vi "Set In Range Trigger.vi"(7 "Trigger Direction":T2, 8 "error in (no error)":errorcluster, 10 "In Range Trigger":T1, 11 "Item Ref in":T3 format="%.0x") -> (0 "error out":errorcluster, 3 "Item Ref out":T3 format="%.0x")   [LabVIEW 2015, in "Waveform Data Logger Shared.lvlib"]
uses:
  Waveform Data Logger Shared.lvlib
  <vilib>/NI Veristand/Custom Device API/Custom Device Item Ref.ctl
  Types/Trigger Direction.ctl
  Types/In Range Trigger.ctl
  Globals/Property Strings.vi
  <vilib>/NI Veristand/Custom Device API/Set Item Property (Double).vi
  <vilib>/NI Veristand/Custom Device API/Set Item Property (Boolean).vi
  <vilib>/NI VeriStand/Custom Device API/Custom Device API.lvlib
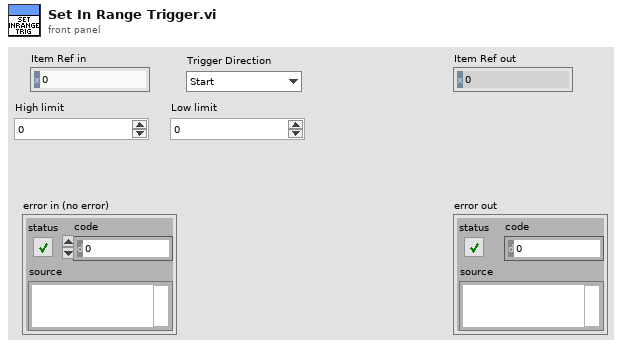
[diagram p1: front panel]
types:
  T1 = typedef "Waveform Data Logger Shared.lvlib/In Range Trigger.ctl" = cluster{"High limit":dbl, "Low limit":dbl, "Invert?":bool}
  T2 = typedef "Waveform Data Logger Shared.lvlib/Trigger Direction.ctl" = enum16{"Start", "Stop"}
  T3 = typedef "Custom Device API.lvlib/Custom Device Item Ref.ctl" = u64
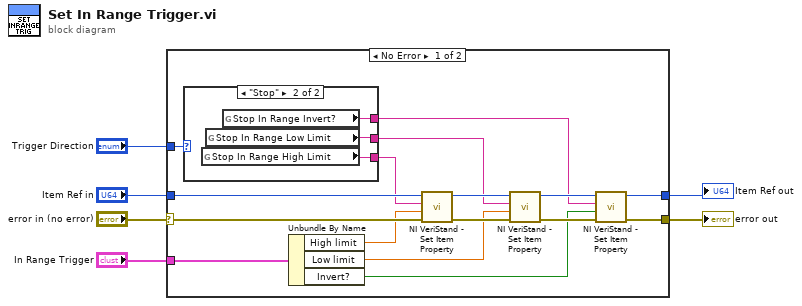
[diagram p0: block diagram]
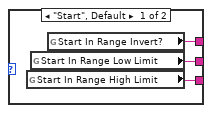
[diagram p2: hidden frame]
diagram:
  n1 = case shown="No Error" "error in (no error)" {
    selector: "error in (no error)" -> [w18 w29]
    tunnel: [w10 w30] -> w6
    tunnel: [w9 w29] -> w5
    tunnel: "Item Ref in" -> [w20 w30]
    tunnel: "In Range Trigger" -> [w19 _]
    tunnel: "Trigger Direction" -> [w17 _]
    frame No Error {
      n2 = case shown="\"Stop\"" w17 {
        tunnel: [w25 w27] -> w13
        tunnel: [w24 w26] -> w14
        tunnel: [w23 w28] -> w7
        frame "Start", Default {
          n3 = global read "Property Strings.vi" "Start In Range High Limit"() -> (w24:string)
          n4 = global read "Property Strings.vi" "Start In Range Low Limit"() -> (w25:string)
          n5 = global read "Property Strings.vi" "Start In Range Invert?"() -> (w23:string)
        }
        frame "Stop" {
          n6 = global read "Property Strings.vi" "Stop In Range High Limit"() -> (w26:string)
          n7 = global read "Property Strings.vi" "Stop In Range Low Limit"() -> (w27:string)
          n8 = global read "Property Strings.vi" "Stop In Range Invert?"() -> (w28:string)
        }
      }
      n9 = Unbundle By Name(w19) -> ("High limit"=w16:dbl, "Low limit"=w15:dbl, "Invert?"=w8:bool)
      n10 = call-poly <vilib>:"NI VeriStand - Set Item Property.vi"("error in (no error)"=w18, "Value"=w16, "Property Name"=w14, "Item Ref in"=w20) -> ("error out"=w22:errorcluster, "Item Ref out"=w21:T3)  [unwired: 5 in, 1 out]
      n11 = call-poly <vilib>:"NI VeriStand - Set Item Property.vi"("error in (no error)"=w22, "Value"=w15, "Property Name"=w13, "Item Ref in"=w21) -> ("error out"=w11:errorcluster, "Item Ref out"=w12:T3)  [unwired: 5 in, 1 out]
      n12 = call-poly <vilib>:"NI VeriStand - Set Item Property.vi"("error in (no error)"=w11, "Value"=w8, "Property Name"=w7, "Item Ref in"=w12) -> ("error out"=w9:errorcluster, "Item Ref out"=w10:T3)  [unwired: 5 in, 1 out]
    }
    frame Error {
    }
  }
  "Item Ref out" <- w6
  "error out" <- w5
